vi "Stop Analyzer VI.vi"(8 "error in (no error)":errorcluster, 9 "Blocking (T)":bool=TRUE, 10 "Process Name":string, 11 "Data in":T1={"Visible Hardware VI"="", "Current Message"={"Source"="", "Destination"="", "Time Stamp"=timestamp(0 s since 1904-01-01), "Command"="", "Data"=variant(string "")}, "Message History"=[], "Hardware"={"Process Cache"=refnum, "Plugins"=[{"Plugin Name"="", "Controller Type"=enum."Invalid", "Control Panel Path"=path "", "Plugin Type"=enum."Optimizer"}, {"Plugin Name"="", "Controller Type"=enum."Invalid", "Control Panel Path"=path "", "Plugin Type"=enum."Optimizer"}, {"Plugin Name"="", "Controller Type"=enum."Invalid", "Control Panel Path"=path "", "Plugin Type"=enum."Optimizer"}, {"Plugin Name"="", "Controller Type"=enum."Invalid", "Control Panel Path"=path "", "Plugin Type"=enum."Optimizer"}]}, "Optimizers"={"Process Cache"=refnum, "Plugins"=[{"Plugin Name"="", "Controller Type"=enum."Invalid", "Control Panel Path"=path "", "Plugin Type"=enum."Optimizer"}, {"Plugin Name"="", "Controller Type"=enum."Invalid", "Control Panel Path"=path "", "Plugin Type"=enum."Optimizer"}, {"Plugin Name"="", "Controller Type"=enum."Invalid", "Control Panel Path"=path "", "Plugin Type"=enum."Optimizer"}], "First parameteres?"=FALSE, "New Parameters"={"Time Stamp"=timestamp(0 s since 1904-01-01), "Names"=[], "Values"=[]}}, "Parameter to Hardware Map"=refnum, "Analyzers"={"Process Cache"=refnum, "Plugins"=[{"Plugin Name"="", "Controller Type"=enum."Invalid", "Control Panel Path"=path "", "Plugin Type"=enum."Optimizer"}, {"Plugin Name"="", "Controller Type"=enum."Invalid", "Control Panel Path"=path "", "Plugin Type"=enum."Optimizer"}, {"Plugin Name"="", "Controller Type"=enum."Invalid", "Control Panel Path"=path "", "Plugin Type"=enum."Optimizer"}, {"Plugin Name"="", "Controller Type"=enum."Invalid", "Control Panel Path"=path "", "Plugin Type"=enum."Optimizer"}]}, "Log Directory"=path "", "Auto Pass Parameters"=FALSE, "Experiment"={"Name"="", "File Path"=path "", "File Extension"="", "File Cluster"={"Hardware List"=[], "Optimizer List"=[], "Analyzer List"=[], "Parameter to Hardware Map"=[]}}, "Main VI Queue"=refnum, "Process Queue References"=[], "Message Queue"=refnum}) -> (0 "error out":errorcluster, 3 "Data out":T1={"Visible Hardware VI"="", "Current Message"={"Source"="", "Destination"="", "Time Stamp"=timestamp(0 s since 1904-01-01), "Command"="", "Data"=variant(string "")}, "Message History"=[], "Hardware"={"Process Cache"=refnum, "Plugins"=[{"Plugin Name"="", "Controller Type"=enum."Invalid", "Control Panel Path"=path "", "Plugin Type"=enum."Optimizer"}, {"Plugin Name"="", "Controller Type"=enum."Invalid", "Control Panel Path"=path "", "Plugin Type"=enum."Optimizer"}, {"Plugin Name"="", "Controller Type"=enum."Invalid", "Control Panel Path"=path "", "Plugin Type"=enum."Optimizer"}, {"Plugin Name"="", "Controller Type"=enum."Invalid", "Control Panel Path"=path "", "Plugin Type"=enum."Optimizer"}]}, "Optimizers"={"Process Cache"=refnum, "Plugins"=[{"Plugin Name"="", "Controller Type"=enum."Invalid", "Control Panel Path"=path "", "Plugin Type"=enum."Optimizer"}, {"Plugin Name"="", "Controller Type"=enum."Invalid", "Control Panel Path"=path "", "Plugin Type"=enum."Optimizer"}, {"Plugin Name"="", "Controller Type"=enum."Invalid", "Control Panel Path"=path "", "Plugin Type"=enum."Optimizer"}], "First parameteres?"=FALSE, "New Parameters"={"Time Stamp"=timestamp(0 s since 1904-01-01), "Names"=[], "Values"=[]}}, "Parameter to Hardware Map"=refnum, "Analyzers"={"Process Cache"=refnum, "Plugins"=[{"Plugin Name"="", "Controller Type"=enum."Invalid", "Control Panel Path"=path "", "Plugin Type"=enum."Optimizer"}, {"Plugin Name"="", "Controller Type"=enum."Invalid", "Control Panel Path"=path "", "Plugin Type"=enum."Optimizer"}, {"Plugin Name"="", "Controller Type"=enum."Invalid", "Control Panel Path"=path "", "Plugin Type"=enum."Optimizer"}, {"Plugin Name"="", "Controller Type"=enum."Invalid", "Control Panel Path"=path "", "Plugin Type"=enum."Optimizer"}]}, "Log Directory"=path "", "Auto Pass Parameters"=FALSE, "Experiment"={"Name"="", "File Path"=path "", "File Extension"="", "File Cluster"={"Hardware List"=[], "Optimizer List"=[], "Analyzer List"=[], "Parameter to Hardware Map"=[]}}, "Main VI Queue"=refnum, "Process Queue References"=[], "Message Queue"=refnum})   [LabVIEW 2020, in "RxnRover.lvlib"]
doc: "Stops the named process, shutting down the subpanel indicator and control panel, removing the entry from the message history cache, and deleting it form the object array. This VI triggers status update events."
uses:
  RxnRover.lvlib
  Controller Array/Controller Array.lvclass
  Type Definitions/Data.ctl
  Parameter to Hardware Map/Parameter to Hardware Map.lvclass
  <userlib>/RxnRover/DynamicReentrant/src/Type Defs/Message.ctl
  Plugin Manager/Plugin Details.ctl
  Controller/Controller Type.ctl
  Plugin Manager/Plugin Types.ctl
  Type Definitions/New Parameters.ctl
  Experiment/Experiment File/Experiment File Cluster.ctl
  Controller/Minimal Controller Cluster.ctl
  Parameter to Hardware Map/Minimal Map.ctl
  Parameter to Hardware Map/Minimal Pair Cluster.ctl
  Controller/Generic Plugin.lvclass
  <userlib>/RxnRover/DynamicReentrant/Dynamic Reentrant.lvlib
  Experiment/Experiment File/Experiment File.lvlib
  Plugin Manager/Plugin Manager.lvlib
panel:
  # "Note: Rxn Rover data control and indicator have been hidden!"
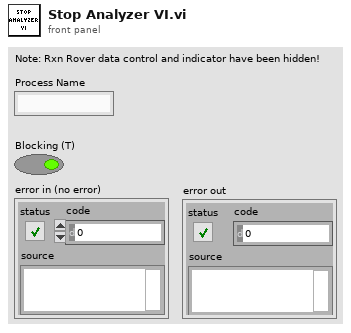
[diagram p1: front panel]
types:
  T1 = typedef "RxnRover.lvlib/Data.ctl" = cluster{"Visible Hardware VI":string, "Current Message":T2, "Message History":string[][], "Hardware":cluster{"Process Cache":refnum<class "Controller Array.lvclass">, "Plugins":T3[]}, "Optimizers":cluster{"Process Cache":refnum<class "Controller Array.lvclass">, "Plugins":T3[], "First parameteres?":bool, "New Parameters":T6}, "Parameter to Hardware Map":refnum<class "Parameter to Hardware Map.lvclass">, "Analyzers":cluster{"Process Cache":refnum<class "Controller Array.lvclass">, "Plugins":T3[]}, "Log Directory":path, "Auto Pass Parameters":bool, "Experiment":cluster{"Name":string, "File Path":path, "File Extension":string, "File Cluster":T7}, "Main VI Queue":refnum<queue>, "Process Queue References":refnum<queue>[], "Message Queue":refnum<queue>}
  T2 = typedef "Dynamic Reentrant.lvlib/Message.ctl" = cluster{"Source":string, "Destination":string, "Time Stamp":timestamp, "Command":string, "Data":variant}
  T3 = typedef "RxnRover.lvlib/Plugin Manager.lvlib/Plugin Details.ctl" = cluster{"Plugin Name":string, "Controller Type":T4, "Control Panel Path":path, "Plugin Type":T5}
  T4 = typedef "RxnRover.lvlib/Generic Plugin.lvclass/Controller Type.ctl" = enum16{"Invalid", "Temperature Controller", "Pump Controller", "Syringe Pump", "Generic Optimizer", "LC Parser"}
  T5 = typedef "RxnRover.lvlib/Plugin Manager.lvlib/Plugin Types.ctl" = enum16{"Invalid", "Optimizer", "Analyzer", "Hardware"}
  T6 = typedef "RxnRover.lvlib/New Parameters.ctl" = cluster{"Time Stamp":timestamp, "Names":string[], "Values":variant[]}
  T7 = typedef "RxnRover.lvlib/Experiment File.lvlib/Experiment File Cluster.ctl" = cluster{"Hardware List":T8[], "Optimizer List":T8[], "Analyzer List":T8[], "Parameter to Hardware Map":T9}
  T8 = typedef "RxnRover.lvlib/Generic Plugin.lvclass/Minimal Controller Cluster.ctl" = cluster{"Name":string, "Controller Type":string, "Control Panel Path":string, "Resource":string}
  T9 = typedef "RxnRover.lvlib/Parameter to Hardware Map.lvclass/Minimal Map.ctl" = T10[]
  T10 = typedef "RxnRover.lvlib/Parameter to Hardware Map.lvclass/Minimal Pair Cluster.ctl" = cluster{"key":string, "values":T8[]}
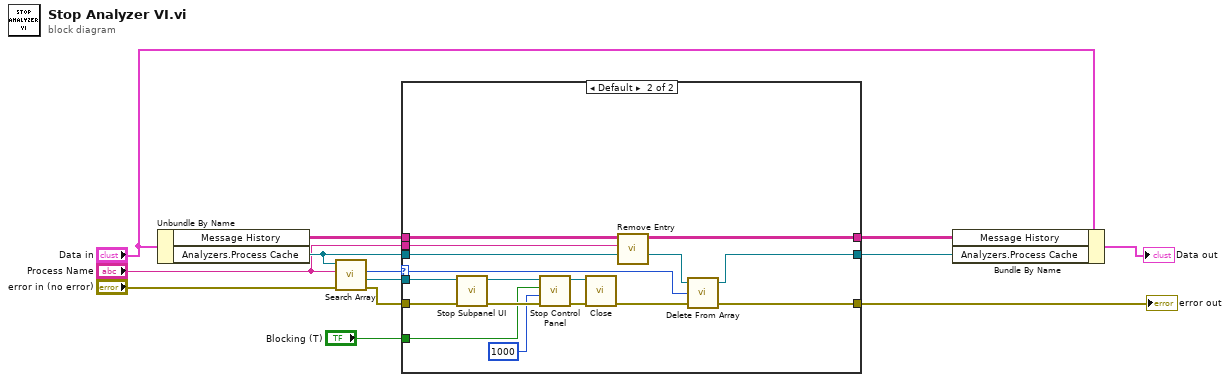
[diagram p0: block diagram]
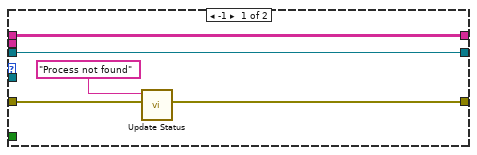
[diagram p2: hidden frame]
diagram:
  n1 = Unbundle By Name("Data in") -> ("Message History"=w7:string[][], "Analyzers.Process Cache"=w8:refnum<class "Controller Array.lvclass">)
  n2 = call "Search Array.vi"("error in (no error)"="error in (no error)", "Search Value"="Process Name", "Controller Array in"=w8) -> ("error out"=w10:errorcluster, "Controller found"=w11:refnum<class "Generic Plugin.lvclass">, "Index of found"=w9:i32)  [unwired: 1 in, 1 out]
  n3 = case shown="Default" w9 {
    selector: w9 -> [_ w30]
    tunnel: [w17 w23] -> w13
    tunnel: w11 -> [_ w33]
    tunnel: w10 -> [w18 w31]
    tunnel: w8 -> [w15 w29]
    tunnel: [w15 w28] -> w3
    tunnel: w7 -> [w14 w27]
    tunnel: "Process Name" -> [_ w26]
    tunnel: [w14 w25] -> w4
    tunnel: "Blocking (T)" -> [_ w24]
    frame -1 {
      n4 = call "Update Status.vi"("error in (no error)"=w18, "Status Bar Text"="Process not found") -> ("error out"=w17:errorcluster)  [unwired: 9 in]
    }
    frame Default {
      n5 = call "Stop Subpanel UI.vi"("error in (no error)"=w31, "Controller in"=w33) -> ("error out"=w34:errorcluster, "Controller out"=w32:refnum<class "Generic Plugin.lvclass">)  [unwired: 8 in]
      n6 = call "Stop Control Panel.vi"("error in (no error)"=w34, "timeout in ms (-1)"=1000, "Blocking (T)"=w24, "controller in"=w32) -> ("error out"=w21:errorcluster, "controller out"=w20:refnum<class "Generic Plugin.lvclass">)  [unwired: 6 in]
      n7 = call "Close.vi"("error in (no error)"=w21, "Plugin in"=w20) -> ("error out"=w19:errorcluster)  [unwired: 9 in]
      n8 = call "Remove Entry.vi"("Source"=w26, "Message History in"=w27) -> ("Message History out"=w25:string[][])  [unwired: 9 in]
      n9 = call "Delete From Array.vi"("error in (no error)"=w19, "index (last elem)"=w30, "Controller Array in"=w29) -> ("error out"=w23:errorcluster, "Controller Array out"=w28:refnum<class "Controller Array.lvclass">)  [unwired: 1 out]
    }
  }
  "error out" <- w13
  n10 = Bundle By Name(cluster="Data in", "Message History"=w4, "Analyzers.Process Cache"=w3) -> (→"Data out":T1)
